vi "MotorEncoder_Init.vi"(2 "error in":errorcluster) -> (0 "error out":errorcluster, 1 "MotorEncoderTasks":refnum<k21>[](array[refnum]))   [LabVIEW 2015]
uses:
  <vilib>/DAQmx/create/channels.llb/DAQmx Create Channel (CI-Position-Angular Encoder).vi
panel:
  in  "pulses per revolution":u32=2048
  in  "units":i32(ring)=10146 items=["Degrees"=10146, "Radians"=10273, "Ticks"=10304, "From Custom Scale"=10065]
  in  "Array":tag[](array[tag])=["PXI1Slot6/ctr0", "PXI1Slot6/ctr1", "PXI1Slot6/ctr2", "PXI1Slot6/ctr3", "PXI1Slot6/ctr4", "PXI1Slot6/ctr5", "PXI1Slot6/ctr6", "PXI1Slot6/ctr7"]
  in  "decoding type":i32(ring)=10092 items=["X1"=10090, "X2"=10091, "X4"=10092, "Two Pulse Counting"=10313]
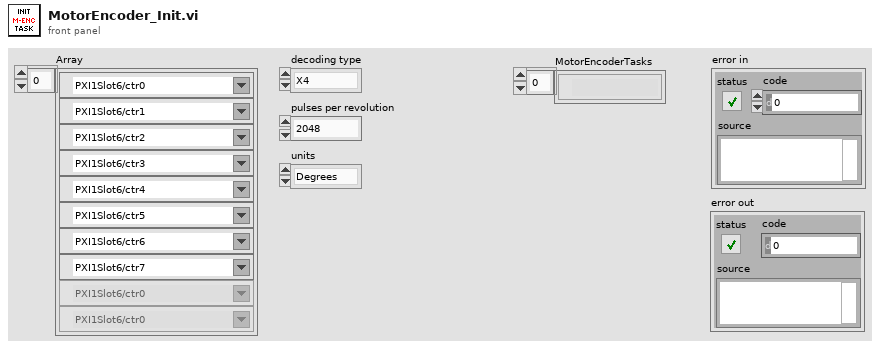
[diagram p1: front panel]
types:
  T1 = cluster{"Input":enum16{"Fr:Cable", "Fr:Motor", "Fr:Sensor"}, "Output":enum16{"To:Cable", "To:Motor", "To:Sensor"}}
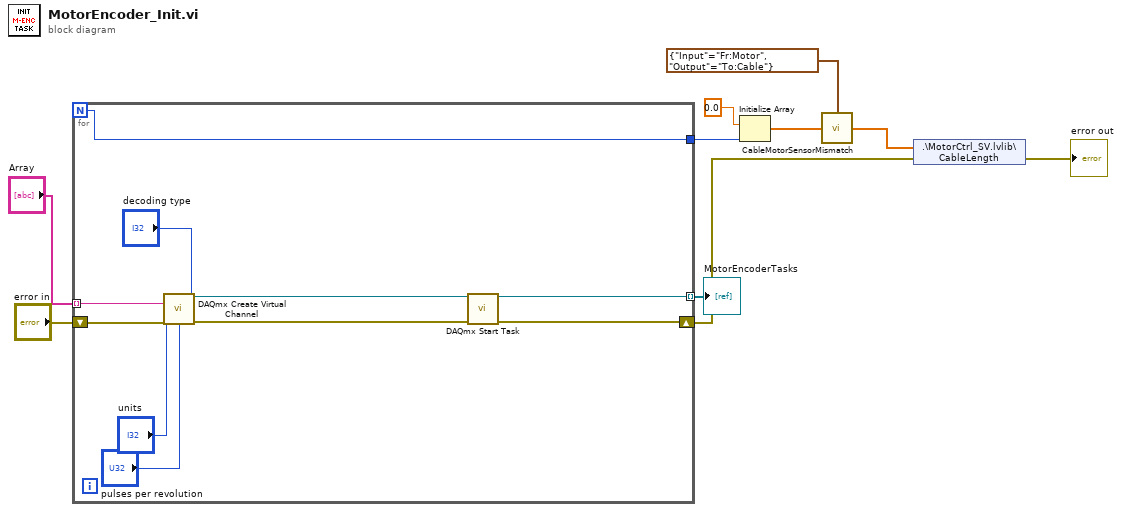
[diagram p0: block diagram]
diagram:
  n1 = for {
    N -> [w11]
    tunnel: "Array" -> [w20] mode=indexing
    tunnel: [w14] -> w9 mode=indexing
    shift-right: [w12] -> w5
    shift-left: "error in" -> [w17]
    tunnel: [w11] -> w7
    n2 = call-poly <vilib>:"DAQmx Create Virtual Channel.vi"("counter"=w20, "decoding type"="decoding type", "units"="units", "error in"=w17, "pulses per revolution"="pulses per revolution") -> ("task out"=w15:refnum<k21>, "error out"=w13:errorcluster)  [unwired: 9 in]
    n3 = call <vilib>:"DAQmx Start Task.vi"("task/channels in"=w15, "error in"=w13) -> ("task out"=w14:refnum<k21>, "error out"=w12:errorcluster)  [unwired: 12 in]
  }
  "MotorEncoderTasks" <- w9
  n4 = Initialize Array(0.0, w7) -> (w3:dbl[])
  n5 = call "CableMotorSensorMismatch.vi"("Conversion"=T1 {"Input"=enum."Fr:Motor", "Output"=enum."To:Cable"}, "Input"=w3) -> ("Output"=w2:dbl[])  [unwired: 2 in]
  n6 = shared-variable ".\\MotorCtrl_SV.lvlib\\CableLength"(w2, error in=w5) -> (error out=→"error out":errorcluster)
